vi "Ch2-Ex2.vi"() -> ()   [LabVIEW 2019]
panel:
  out "Time between executions (Seconds)":dbl
  in  "ms to Wait":dbl
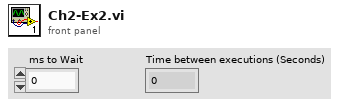
[diagram p1: front panel]
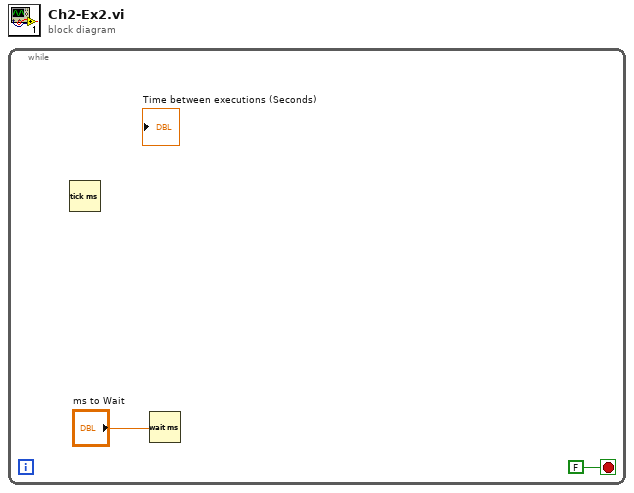
[diagram p0: block diagram]
diagram:
  n1 = while {
    stop <- FALSE stop-if-true
    n2 = Tick Count (ms)() -> ()  [unwired: 1 out]
    n3 = Wait (ms)(milliseconds to wait="ms to Wait") -> ()  [unwired: 1 out]
  }
